vi "CRYASIO Global.vi"() -> ()   [LabVIEW 2013]
panel:
  in  "Inited ASIO Driver Name":string
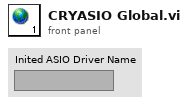
[diagram p1: front panel]
diagram:
